vi "Stop Core.vi"(10 "final error code":i32, 11 "Cli in":refnum<class "Cli.lvclass">) -> (3 "Cli out":refnum<class "Cli.lvclass">)   [LabVIEW 2022 SP3, in "Cli.lvlib" / "Cli.lvclass"]
doc: "(<B>Filename</B>: Actor Framework.lvlib:Actor.lvclass:Stop Core.vi)\n\nDefines what the actor does before it stops. Use the <B>final error code</B> input to determine whether the actor shut down in response to an error.\n\nBy default, this method does nothing. A descendant class may override it to define behavior, such as shutting down any processes the actor initiated in its override of the Actor Core method."
uses:
  Cli.lvclass
  Cli.lvclass/Cli.ctl
  ArgumentParser/Source/ArgumentParser/ArgumentParser.lvclass
  LoggingActor/Source/LoggingActor/LoggingActor/LoggingActor.lvclass
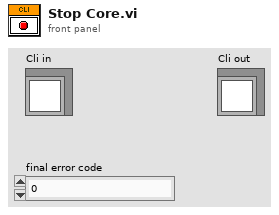
[diagram p1: front panel]
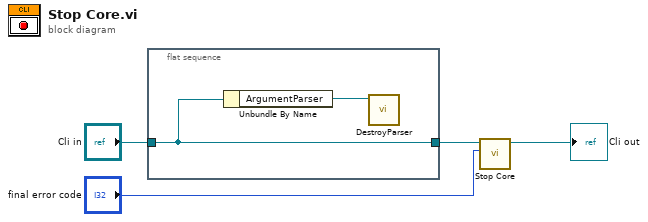
[diagram p0: block diagram]
diagram:
  n1 = flat-sequence {
    tunnel: "Cli in" -> [w5]
    tunnel: [w5] -> w1
    frame #0 {
      n2 = Unbundle By Name(w5) -> ("ArgumentParser"=w6:refnum<class "ArgumentParser.lvclass">)
      n3 = call-dynamic "DestroyParser.vi"("ArgumentParser in"=w6) -> ()  [unwired: 10 in, 1 out]
    }
  }
  n4 = call-parent "Stop Core.vi"("final error code"="final error code", "LoggingActor in"=w1) -> ("LoggingActor out"=→"Cli out":refnum<class "Cli.lvclass">)  [unwired: 9 in]
